vi "Request UI Display.vi"(6 "wait for reply (T)":bool=TRUE, 8 "error in (no error)":errorcluster, 10 "Scenario":T1) -> (0 "error out":errorcluster, 3 "Accept?":bool)   [LabVIEW 2020, in "DBModule.lvlib"]
doc: "Requests the module to display its UI as specified in <b>Scenario</b>:\n\"managed\" => in the UI Manager's subpanel\n\"stand-alone\" => as a separate window\n____\nHAMPEL SOFTWARE ENGINEERING v2.6.0 (2023-12-19 10:54)"
uses:
  DBModule.lvlib
  Libraries/hse-libraries/Source/hse-dqmh/Controls/Module Display Scenarios.ctl
  Request UI Display Argument--cluster.ctl
  Request UI Display (Reply Payload)--cluster.ctl
  Libraries/hse-libraries/Source/hse-dqmh/hse-dqmh.lvlib
panel:
  out "timed out?":bool
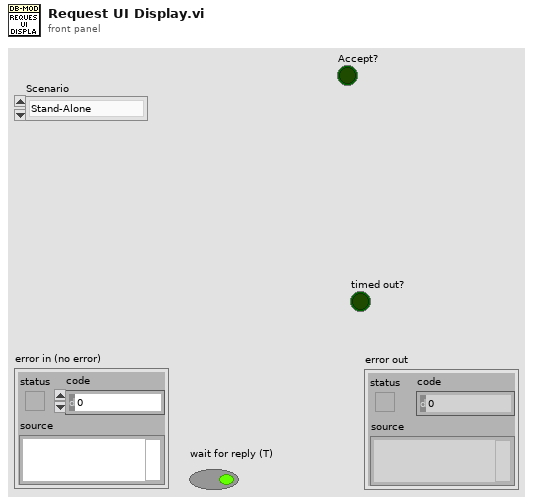
[diagram p1: front panel]
types:
  T1 = typedef "hse-dqmh.lvlib/Module Display Scenarios.ctl" = enum16{"Stand-Alone", "Managed"}
  T2 = typedef "DBModule.lvlib/Request UI Display Argument--cluster.ctl" = cluster{"Scenario":T1, "Wait Notifier":refnum<notifier>, "wait for reply":bool}
  T3 = typedef "DBModule.lvlib/Request Events--cluster.ctl" = cluster{"Stop Module":refnum<user-event>, "Show Panel":refnum<user-event>, "Hide Panel":refnum<user-event>, "Get Module Execution Status":refnum<user-event>, "Show Diagram":refnum<user-event>, "Configure":refnum<user-event>, "Prepare":refnum<user-event>, "Request UI Display":refnum<user-event>, "Start and Configure DB_Connector":refnum<user-event>}
  T4 = typedef "DBModule.lvlib/Request UI Display (Reply Payload)--cluster.ctl" = cluster{"Accept?":bool, "Request UI Display_error":errorcluster}
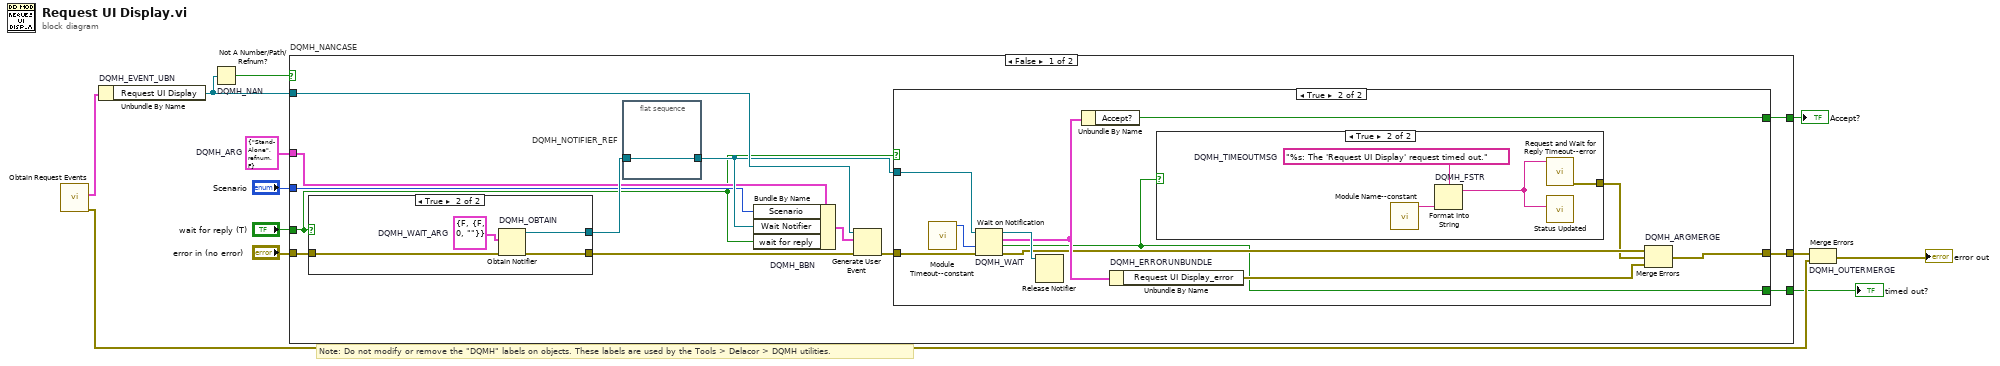
[diagram p0: block diagram]
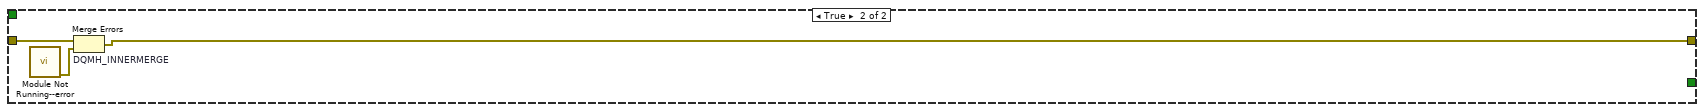
[diagram p5: hidden frame]
diagram:
  w7 = T2 {"Scenario"=enum."Stand-Alone", "Wait Notifier"=refnum, "wait for reply"=FALSE}  # DQMH_ARG
  # "Note: Do not modify or remove the \"DQMH\" labels on objects. These labels are used by the Tools > Delacor > DQMH utilities."
  n1 = call "Obtain Request Events.vi"() -> ("error out"=w4:errorcluster, "DBModule Request Events"=w3:T3)  [unwired: 10 in]
  n2 = Unbundle By Name "DQMH_EVENT_UBN"(w3) -> ("Request UI Display"=w10:refnum<user-event>)
  n3 = Not A Number/Path/Refnum? "DQMH_NAN"(number/path/refnum=w10) -> (NaN/Path/Refnum?=w9:bool)
  n4 = case "DQMH_NANCASE" shown="False" w9 {
    tunnel: "error in (no error)" -> [w25 w50]
    tunnel: w10 -> [w23 _]
    tunnel: [w21 w49] -> w8
    tunnel: w7 -> [w17 _]
    tunnel: "Scenario" -> [w16 _]
    tunnel: "wait for reply (T)" -> [w15 _]
    tunnel: [w14 _] -> w2
    tunnel: [w13 _] -> w1
    frame False {
      n5 = case shown="True" w15 {
        tunnel: w25 -> [w43 w47]
        tunnel: [w43 w46] -> w22
        tunnel: [_ w44] -> w19
        frame False {
        }
        frame True {
          w45 = T4 {"Accept?"=FALSE, "Request UI Display_error"={"status"=FALSE, "code"=0, "source"=""}}  # DQMH_WAIT_ARG
          n6 = Obtain Notifier "DQMH_OBTAIN"(notification data type=w45, error in (no error)=w47) -> (notifier out=w44:refnum<notifier>, error out=w46:errorcluster)  [unwired: 2 in, 1 out]
        }
      }
      n7 = flat-sequence "DQMH_NOTIFIER_REF" {
        tunnel: w19 -> [w26]
        tunnel: [w26] -> w18
        frame #0 {
        }
      }
      n8 = Bundle By Name "DQMH_BBN"(cluster=w17, "Scenario"=w16, "Wait Notifier"=w18, "wait for reply"=w15) -> (w20:T2)
      n9 = Generate User Event(user event=w23, event data cluster=w20, error in=w22) -> (error out=w24:errorcluster)  [unwired: 1 in, 1 out]
      n10 = case shown="True" w15 {
        tunnel: w24 -> [w27 w38]
        tunnel: w18 -> [_ w37]
        tunnel: [w27 w35] -> w21
        tunnel: [_ w31] -> w14
        tunnel: [_ w28] -> w13
        frame False {
        }
        frame True {
          n11 = call "Module Timeout--constant.vi"() -> ("Module Timeout"=w33:i32)  [unwired: 11 in]
          n12 = Wait on Notification "DQMH_WAIT"(notifier=w37, timeout in ms (-1)=w33, error in (no error)=w38) -> (notifier out=w36:refnum<notifier>, notification=w32:T4, timed out?=w28:bool, error out=w30:errorcluster)  [unwired: 1 in]
          n13 = Release Notifier(notifier=w36) -> ()  [unwired: 2 in, 3 out]
          n14 = Unbundle By Name(w32) -> ("Accept?"=w31:bool)
          n15 = Unbundle By Name "DQMH_ERRORUNBUNDLE"(w32) -> ("Request UI Display_error"=w34:errorcluster)
          n16 = case shown="True" w28 {
            tunnel: [_ w39] -> w29
            frame False {
            }
            frame True {
              w42 = "%s: The 'Request UI Display' request timed out."  # DQMH_TIMEOUTMSG
              n17 = call "Module Name--constant.vi"() -> ("Module Name"=w41:string)  [unwired: 11 in]
              n18 = Format Into String "DQMH_FSTR"(format string=w42, w41) -> (resulting string=w40:string)  [unwired: 2 in, 1 out]
              n19 = call "Request and Wait for Reply Timeout--error.vi"("Error Message"=w40) -> ("error out"=w39:errorcluster)  [unwired: 10 in]
              n20 = call "Status Updated.vi"("Status"=w40) -> ()  [unwired: 10 in, 1 out]
            }
          }
          n21 = Merge Errors "DQMH_ARGMERGE"(w30, w29, w34) -> (w35:errorcluster)
        }
      }
    }
    frame True {
      n22 = call "Module Not Running--error.vi"() -> ("error out"=w48:errorcluster)  [unwired: 11 in]
      n23 = Merge Errors "DQMH_INNERMERGE"(w50, w48) -> (w49:errorcluster)
    }
  }
  "Accept?" <- w2
  "timed out?" <- w1
  n24 = Merge Errors "DQMH_OUTERMERGE"(w8, w4) -> (→"error out":errorcluster)
